vi "ep_Write Voltage Sensitivity (Multiple Lines).vi"(8 "error in (no error)":errorcluster, 10 "voltage sensitivity (multiline)":T1[](array[typedef]), 11 "system info in":refnum<class "EP System Info.lvclass">) -> (0 "error out":errorcluster, 3 "system info out":refnum<class "EP System Info.lvclass">)   [LabVIEW 2014, in "NI_EP_Power Quality.lvlib" / "EP System Info.lvclass"]
uses:
  <vilib>/addons/Electrical Power/PQ/Common/Classes/System Info/EP System Info.lvclass
  <vilib>/addons/Electrical Power/PQ/Common/Controls/ep_Channel Sensitivity.ctl
  <vilib>/addons/Electrical Power/PQ/Common/Classes/System Info/EP System Info.lvclass/EP System Info.ctl
  <vilib>/addons/Electrical Power/PQ/NI_EP_Power Quality.lvlib
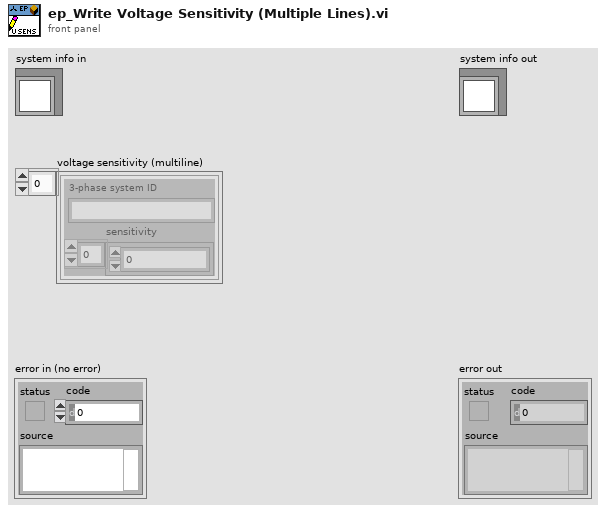
[diagram p1: front panel]
types:
  T1 = typedef "NI_EP_Power Quality.lvlib/ep_Channel Sensitivity.ctl" = cluster{"3-phase system ID":string, "sensitivity":dbl[]}
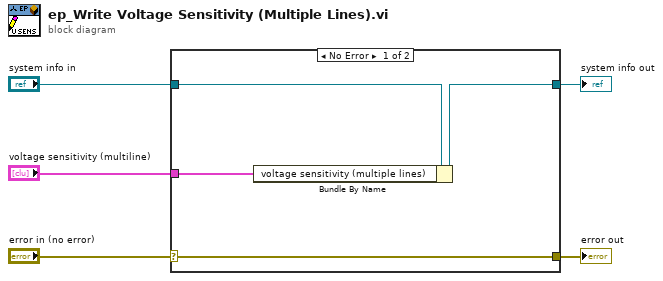
[diagram p0: block diagram]
diagram:
  n1 = case shown="No Error" "error in (no error)" {
    selector: "error in (no error)" -> [w9 w10]
    tunnel: [w9 w10] -> w4
    tunnel: [w7 w11] -> w2
    tunnel: "system info in" -> [w8 w11]
    tunnel: "voltage sensitivity (multiline)" -> [w6 _]
    frame No Error {
      n2 = Bundle By Name(cluster=w8, "voltage sensitivity (multiple lines)"=w6) -> (w7:refnum<class "EP System Info.lvclass">)
    }
    frame Error {
    }
  }
  "error out" <- w4
  "system info out" <- w2
